vi "test_TxUDP-RxUDP - Multiple Boards - 160 Channels.vi"(8 "error in":errorcluster, 11 "reference in":refnum<class "AIM ARINC 664 Loopback.lvclass">) -> (0 "error out":errorcluster, 3 "reference out":refnum<class "AIM ARINC 664 Loopback.lvclass">)   [LabVIEW 2020, in "AIM ARINC 664 Loopback.lvclass"]
uses:
  AIM ARINC 664 Loopback.lvclass
  C:/Program Files (x86)/National Instruments/LabVIEW 2020/vi.lib/NI/VeriStand Custom Device Testing Tools/VeriStandTestCase/VeriStandTestCase.lvclass
  AIM ARINC 664 Loopback.lvclass/AIM ARINC 664 Loopback.ctl
  NationalInstruments.VeriStand.SystemDefinitionAPI
  b47c41b5-a02e-49d5-b852-4e28f097d7ad.vi
  1d1f42d9-2e54-4610-b77a-bc9f79ee4e8b.vi
  c995a650-bbae-43dd-bdca-b2725b3d2010.vi
  <vilib>/addons/_JKI Toolkits/VI Tester/TestCase.llb/TestCase.lvclass
  6a3dd3ed-914d-4d14-bf18-724521aa5e28.vi
  Scripting/AIM ARINC 664 Scripting.lvlib
  <vilib>/NI/VeriStand Custom Device Testing Tools/VeriStandTestCase/VeriStandTestCase.lvclass
  8abe1e9f-12f7-4d29-bb0e-ea5e1950c3f4.vi
  C:/Program Files (x86)/National Instruments/LabVIEW 2020/vi.lib/addons/_JKI Toolkits/VI Tester/TestCase.llb/TestCase.lvclass
panel:
  in  "# of channels":i32=16
  out "resulting string 2":string
  out "resulting string":string
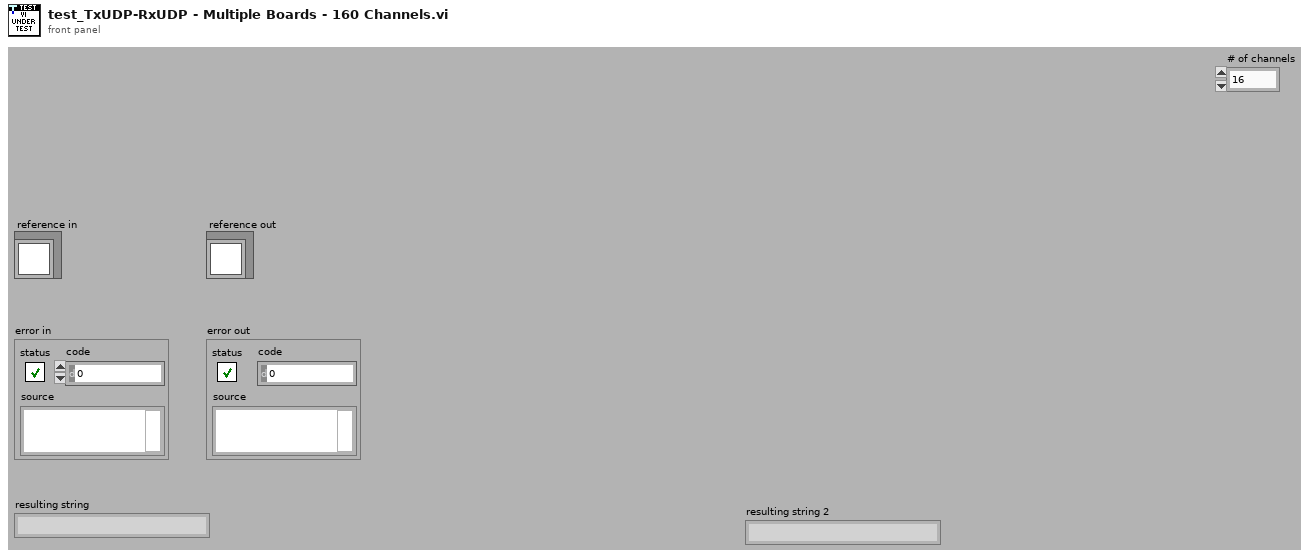
[diagram p1: front panel]
types:
  T1 = typedef "Custom Device API.lvlib/Custom Device Item Ref.ctl" = u64
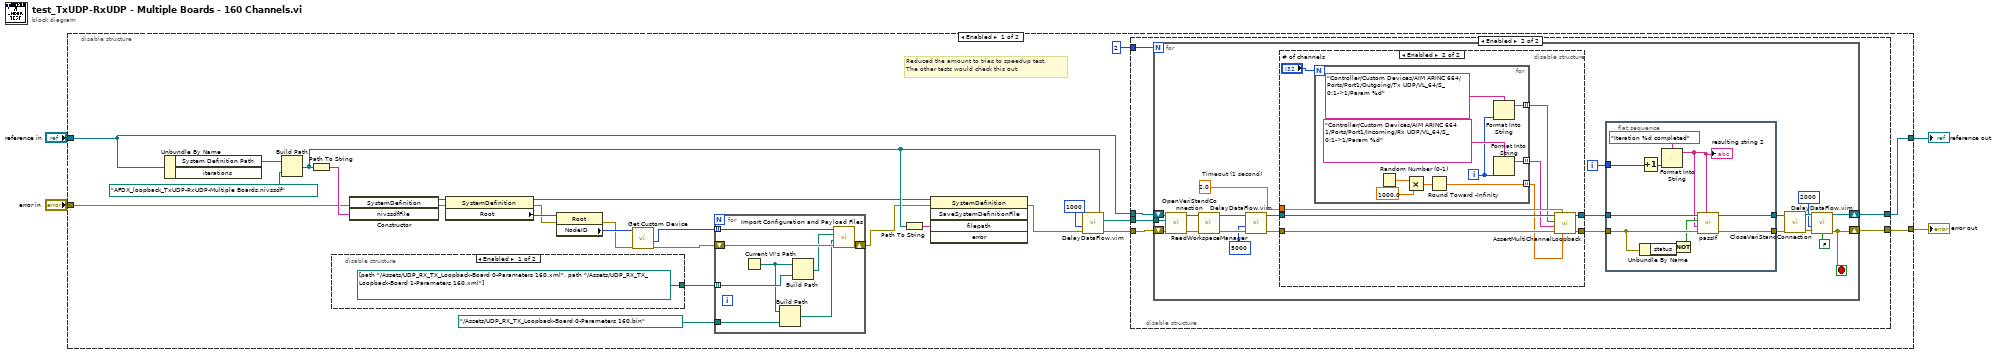
[diagram p0: block diagram]
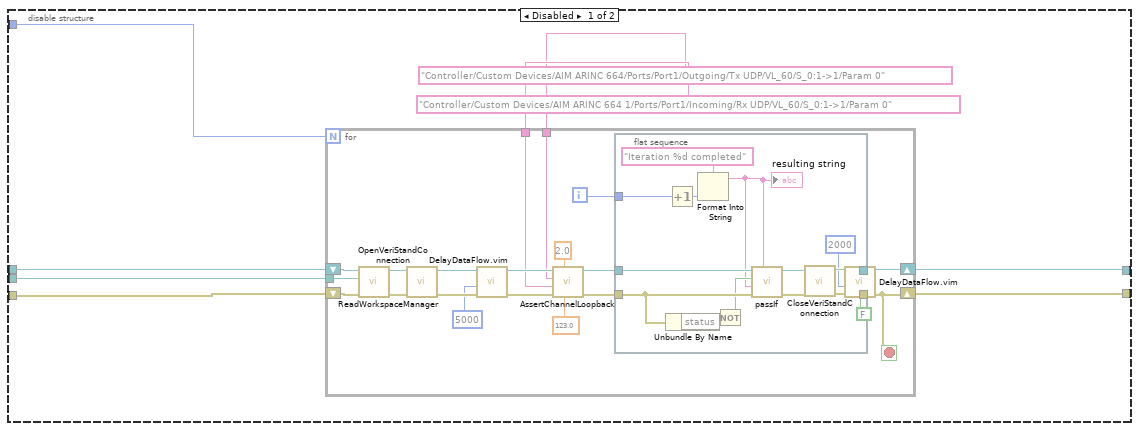
[diagram p2: hidden frame]
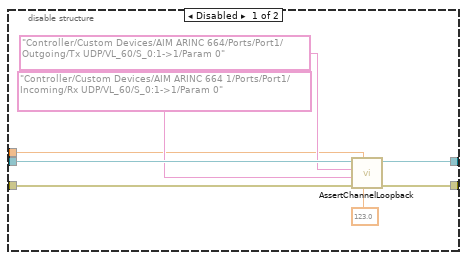
[diagram p3: hidden frame]
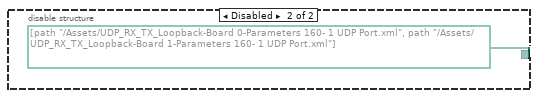
[diagram p4: hidden frame]
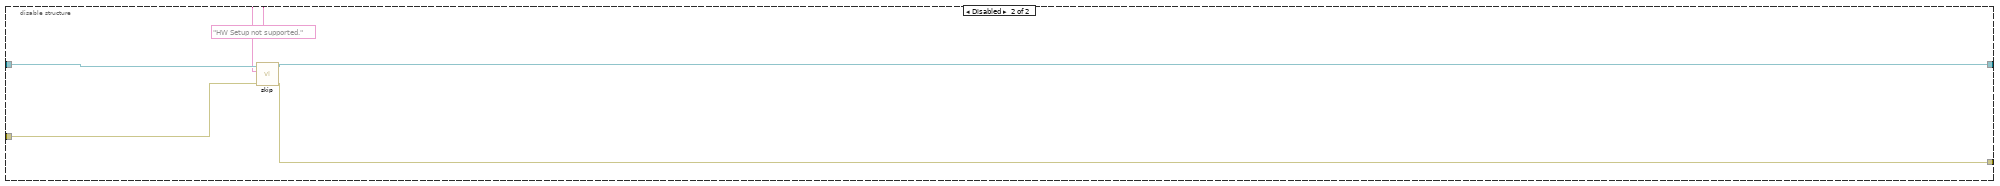
[diagram p5: hidden frame]
diagram:
  n1 = disable-structure shown="Enabled" {
    disable-tunnel: "reference in" -> [w12 w147]
    disable-tunnel: "error in" -> [w11 w146]
    disable-tunnel: [w7 w145] -> w2
    disable-tunnel: [w6 w144] -> w1
    frame Enabled {
      # "Reduced the amount to tries to speedup test.\nThe other tests would check this out."
      n2 = Unbundle By Name(w12) -> ("System Definition Path"=w29:path)  [unwired: 1 out]
      n3 = Build Path(base path=w29, name or relative path=path "AFDX_loopback_TxUDP-RxUDP-Multiple Boards.nivssdf") -> (appended path=w26:path)
      n4 = Path To String(path=w26) -> (string=w27:string)
      n5 = disable-structure shown="Enabled" {
        disable-tunnel: [path[] [path "../Assets/UDP_RX_TX_Loopback-Board 0-Parameters 160.xml", path "../Assets/UDP_RX_TX_Loopback-Board 1-Parameters 160.xml"] path[] [path "../Assets/UDP_RX_TX_Loopback-Board 0-Parameters 160- 1 UDP Port.xml", path "../Assets/UDP_RX_TX_Loopback-Board 1-Parameters 160- 1 UDP Port.xml"]] -> w9
        frame Enabled {
        }
        frame Disabled {
        }
      }
      n6 = constructor class="SystemDefinition"(error in=w11, "nivssdfFile"=w27) -> (reference out=w25:refnum<k24>, error out=w23:errorcluster)  [unwired: 2 in, 2 out]
      n7 = property class="SystemDefinition"(reference=w25, error in=w23) -> (reference out=w20:refnum<k24>, error out=w22:errorcluster, "Root"=w24:refnum<k24>)
      n8 = property class="Root"(reference=w24, error in=w22) -> (error out=w17:errorcluster, "NodeID"=w18:u64)  [unwired: 1 out]
      n9 = call "Get Custom Device.vi"("error in"=w17, "custom device ref in"=w18) -> ("error out"=w16:errorcluster, "Item Refs"=w10:T1[])  [unwired: 5 in, 3 out]
      n10 = for {
        shift-right: [w141] -> w21
        shift-left: w16 -> [w142]
        tunnel: w9 -> [w138] mode=indexing
        tunnel: w10 -> [w137] mode=indexing
        tunnel: path "../Assets/UDP_RX_TX_Loopback-Board 0-Parameters 160.bin" -> [w135]
        n11 = Current VI's Path() -> (path=w136:path)
        n12 = Build Path(base path=w136, name or relative path=w135) -> (appended path=w140:path)
        n13 = Build Path(base path=w136, name or relative path=w138) -> (appended path=w139:path)
        n14 = call "Import Configuration and Payload Files.vi"("error in"=w142, "payload file path"=w140, "parameters configuration file path"=w139, "custom device ref"=w137) -> ("error out"=w141:errorcluster)  [unwired: 6 in, 1 out]
      }
      n15 = Path To String(path=w26) -> (string=w19:string)
      n16 = invoke class="SystemDefinition" method="SaveSystemDefinitionFile"(reference=w20, error in=w21, "filepath"=w19) -> (error out=w15:errorcluster)  [unwired: 2 in, 4 out]
      n17 = call "DelayDataFlow.vim"("value in"=w15, "milliseconds to wait"=u32 1000) -> ("value out"=w14:errorcluster)  [unwired: 2 in, 1 out]
      n18 = disable-structure shown="Enabled" {
        disable-tunnel: [w37 w72] -> w7
        disable-tunnel: w26 -> [w36 w75]
        disable-tunnel: w14 -> [w35 w74]
        disable-tunnel: w12 -> [w32 w76]
        disable-tunnel: [w31 w73] -> w6
        disable-tunnel: 2 -> [w30 w71]
        frame Disabled {
          n19 = for {
            N: w30 -> [_]
            tunnel: w36 -> [w53]
            shift-right: [w58] -> w31
            shift-left: w32 -> [w60]
            shift-right: [w38] -> w37
            shift-left: w35 -> [w54]
            tunnel: "Controller/Custom Devices/AIM ARINC 664 1/Ports/Port1/Incoming/Rx UDP/VL_60/S_0:1->1/Param 0" -> [w40]
            tunnel: "Controller/Custom Devices/AIM ARINC 664/Ports/Port1/Outgoing/Tx UDP/VL_60/S_0:1->1/Param 0" -> [w39]
            i -> [w42]
            stop <- w38 stop-if-true
            n20 = call-dynamic "OpenVeriStandConnection.vi"("error in (no error)"=w54, "System Definition File"=w53, "VeriStand Test Case in"=w60) -> ("error out"=w59:errorcluster, "VeriStand Test Case out"=w57:refnum<class "AIM ARINC 664 Loopback.lvclass">)  [unwired: 6 in, 1 out]
            n21 = call-dynamic "ReadWorkspaceManager.vi"("error in (no error)"=w59, "VeriStand Test Case in"=w57) -> ("error out"=w56:errorcluster, "VeriStand Test Case out"=w51:refnum<class "AIM ARINC 664 Loopback.lvclass">)  [unwired: 7 in, 1 out]
            n22 = call "DelayDataFlow.vim"("value in"=w56, "milliseconds to wait"=u32 5000) -> ("value out"=w52:errorcluster)  [unwired: 2 in, 1 out]
            n23 = call <vilib>:"AssertChannelLoopback.vi"("Value"=123.0, "Timeout (1 second)"=2.0, "error in (no error)"=w52, "Read Channel"=w40, "Write Channel"=w39, "VeriStand Test Case in"=w51) -> ("error out"=w43:errorcluster, "VeriStand Test Case out"=w41:refnum<class "AIM ARINC 664 Loopback.lvclass">)  [unwired: 4 in]
            n24 = flat-sequence {
              tunnel: [w70] -> w45
              tunnel: [w69] -> w44
              tunnel: w43 -> [w68]
              tunnel: w42 -> [w64]
              tunnel: w41 -> [w62]
              frame #0 {
                n25 = Unbundle By Name(w68) -> ("status"=w67:bool)
                n26 = Increment(x=w64) -> (x+1=w63:i32)
                n27 = Format Into String(format string="Iteration %d completed", w63) -> (resulting string=w61:string)  [unwired: 2 in, 1 out]
                "resulting string" <- w61
                n28 = Not(x=w67) -> (.not. x?=w66:bool)
                n29 = call-dynamic "passIf.vi"("custom report message (\"\")"=w61, "error in (no error)"=w68, "message (\"\")"=w61, "pass"=w66, "TestCase in"=w62) -> ("error out"=w69:errorcluster, "TestCase out"=w70:refnum<class "AIM ARINC 664 Loopback.lvclass">)  [unwired: 5 in]
              }
            }
            n30 = call-dynamic "CloseVeriStandConnection.vi"("error in (no error)"=w44, "VeriStand Test Case in"=w45) -> ("error out"=w48:errorcluster, "VeriStand Test Case out"=w58:refnum<class "AIM ARINC 664 Loopback.lvclass">)  [unwired: 8 in]
            n31 = call "DelayDataFlow.vim"("value in"=w48, "milliseconds to wait"=u32 2000, "no delay on error (T)"=FALSE) -> ("value out"=w38:errorcluster)  [unwired: 1 in, 1 out]
          }
        }
        frame Enabled {
          n32 = for {
            N: w71 -> [_]
            tunnel: w75 -> [w89]
            shift-right: [w94] -> w73
            shift-left: w76 -> [w96]
            shift-right: [w78] -> w72
            shift-left: w74 -> [w90]
            i -> [w80]
            stop <- w78 stop-if-true
            w77 = 2.0  # Timeout (1 second)
            n33 = call-dynamic "OpenVeriStandConnection.vi"("error in (no error)"=w90, "System Definition File"=w89, "VeriStand Test Case in"=w96) -> ("error out"=w95:errorcluster, "VeriStand Test Case out"=w93:refnum<class "AIM ARINC 664 Loopback.lvclass">)  [unwired: 6 in, 1 out]
            n34 = call-dynamic "ReadWorkspaceManager.vi"("error in (no error)"=w95, "VeriStand Test Case in"=w93) -> ("error out"=w92:errorcluster, "VeriStand Test Case out"=w87:refnum<class "AIM ARINC 664 Loopback.lvclass">)  [unwired: 7 in, 1 out]
            n35 = call "DelayDataFlow.vim"("value in"=w92, "milliseconds to wait"=u32 5000) -> ("value out"=w88:errorcluster)  [unwired: 2 in, 1 out]
            n36 = disable-structure shown="Enabled" {
              disable-tunnel: w88 -> [w104 w110]
              disable-tunnel: w87 -> [w103 w113]
              disable-tunnel: [w101 w111] -> w81
              disable-tunnel: [w100 w112] -> w79
              disable-tunnel: w77 -> [w97 w109]
              frame Disabled {
                n37 = call <vilib>:"AssertChannelLoopback.vi"("Value"=123.0, "Timeout (1 second)"=w97, "error in (no error)"=w104, "Read Channel"="Controller/Custom Devices/AIM ARINC 664 1/Ports/Port1/Incoming/Rx UDP/VL_60/S_0:1->1/Param 0", "Write Channel"="Controller/Custom Devices/AIM ARINC 664/Ports/Port1/Outgoing/Tx UDP/VL_60/S_0:1->1/Param 0", "VeriStand Test Case in"=w103) -> ("error out"=w101:errorcluster, "VeriStand Test Case out"=w100:refnum<class "AIM ARINC 664 Loopback.lvclass">)  [unwired: 4 in]
              }
              frame Enabled {
                n38 = for {
                  N: "# of channels" -> [_]
                  tunnel: [w119] -> w105 mode=indexing
                  tunnel: [w115] -> w107 mode=indexing
                  tunnel: [w114] -> w106 mode=indexing
                  i -> [w116]
                  n39 = Random Number (0-1)() -> (number: 0 to 1=w122:dbl)
                  n40 = Multiply(x=w122, y=1000.0) -> (x*y=w120:dbl)
                  n41 = Round Toward -Infinity(1:w120) -> (0:w119:dbl)
                  n42 = Format Into String(format string="Controller/Custom Devices/AIM ARINC 664/Ports/Port1/Outgoing/Tx UDP/VL_64/S_0:1->1/Param %d", w116) -> (resulting string=w115:string)  [unwired: 2 in, 1 out]
                  n43 = Format Into String(format string="Controller/Custom Devices/AIM ARINC 664 1/Ports/Port1/Incoming/Rx UDP/VL_64/S_0:1->1/Param %d", w116) -> (resulting string=w114:string)  [unwired: 2 in, 1 out]
                }
                n44 = call <vilib>:"AssertMultiChannelLoopback.vi"("Values"=w105, "Timeout (1 second)"=w109, "error in (no error)"=w110, "Read Channels"=w106, "Write Channels"=w107, "VeriStand Test Case in"=w113) -> ("error out"=w111:errorcluster, "VeriStand Test Case out"=w112:refnum<class "AIM ARINC 664 Loopback.lvclass">)  [unwired: 4 in]
              }
            }
            n45 = flat-sequence {
              tunnel: [w132] -> w83
              tunnel: [w131] -> w82
              tunnel: w81 -> [w130]
              tunnel: w80 -> [w126]
              tunnel: w79 -> [w124]
              frame #0 {
                n46 = Unbundle By Name(w130) -> ("status"=w129:bool)
                n47 = Increment(x=w126) -> (x+1=w125:i32)
                n48 = Format Into String(format string="Iteration %d completed", w125) -> (resulting string=w123:string)  [unwired: 2 in, 1 out]
                "resulting string 2" <- w123
                n49 = Not(x=w129) -> (.not. x?=w128:bool)
                n50 = call-dynamic "passIf.vi"("custom report message (\"\")"=w123, "error in (no error)"=w130, "message (\"\")"=w123, "pass"=w128, "TestCase in"=w124) -> ("error out"=w131:errorcluster, "TestCase out"=w132:refnum<class "AIM ARINC 664 Loopback.lvclass">)  [unwired: 5 in]
              }
            }
            n51 = call-dynamic "CloseVeriStandConnection.vi"("error in (no error)"=w82, "VeriStand Test Case in"=w83) -> ("error out"=w86:errorcluster, "VeriStand Test Case out"=w94:refnum<class "AIM ARINC 664 Loopback.lvclass">)  [unwired: 8 in]
            n52 = call "DelayDataFlow.vim"("value in"=w86, "milliseconds to wait"=u32 2000, "no delay on error (T)"=FALSE) -> ("value out"=w78:errorcluster)  [unwired: 1 in, 1 out]
          }
        }
      }
    }
    frame Disabled {
      n53 = call <vilib>:"skip.vi"("error in (no error)"=w146, "skipMessage"="HW Setup not supported.", "TestCase in"=w147) -> ("error out"=w145:errorcluster, "TestCase out"=w144:refnum<class "AIM ARINC 664 Loopback.lvclass">)  [unwired: 7 in]
    }
  }
  "error out" <- w2
  "reference out" <- w1
